vi "KDC101_Init.vi"(8 "error in (no error)":errorcluster caption="entrée d'erreur (pas d'erreur)", 11 "serialNo":string) -> (0 "error out":errorcluster caption="sortie d'erreur", 1 "Connected":bool, 2 "DevManRef":refnum<k24>, 3 "KCubeDCServoRef":refnum<k24>, 4 "SpeedSettings":T1, 5 "IsHomed":bool)   [LabVIEW 2019]
doc: "Utilisez ce modèle pour construire un VI à utiliser en tant que sous-VI."
uses:
  C:/Program Files (x86)/National Instruments/LabVIEW 2019/user.lib/ThorKDC101/Kinesis_with_LabVIEW_Examples_LV12 - v3/Thorlabs.MotionControl.DeviceManagerCLI.dll
  Kinesis_with_LabVIEW_Examples_LV12 - v3/Thorlabs.MotionControl.DeviceManagerCLI.dll
  C:/Program Files (x86)/National Instruments/LabVIEW 2019/user.lib/ThorKDC101/Kinesis_with_LabVIEW_Examples_LV12 - v3/ThorLabs.MotionControl.KCube.DCServoCLI.dll
  Kinesis_with_LabVIEW_Examples_LV12 - v3/ThorLabs.MotionControl.KCube.DCServoCLI.dll
  C:/Program Files (x86)/National Instruments/LabVIEW 2019/user.lib/ThorKDC101/Kinesis_with_LabVIEW_Examples_LV12 - v3/Thorlabs.MotionControl.GenericMotorCLI.dll
  Kinesis_with_LabVIEW_Examples_LV12 - v3/Thorlabs.MotionControl.GenericMotorCLI.dll
panel:
  out "MinVelocity":dbl
  out "MaxVelocity":dbl
  out "Acceleration":dbl
  out "array":string[](array[string])=["", "", "", "", "", "", "", "", "", "", " "]
  out "Capacity":i32
  out "Count":i32
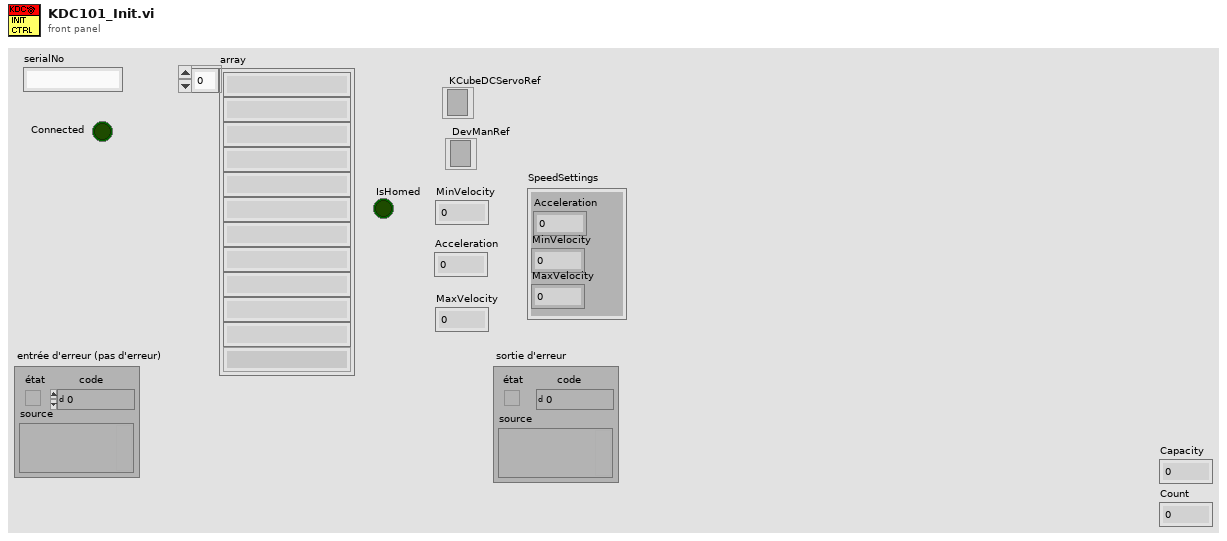
[diagram p1: front panel]
types:
  T1 = cluster{"Acceleration":dbl, "MinVelocity":dbl, "MaxVelocity":dbl}
  T2 = cluster{"Acceleration":dbl, "MaxVelocity":dbl, "MinVelocity":dbl}
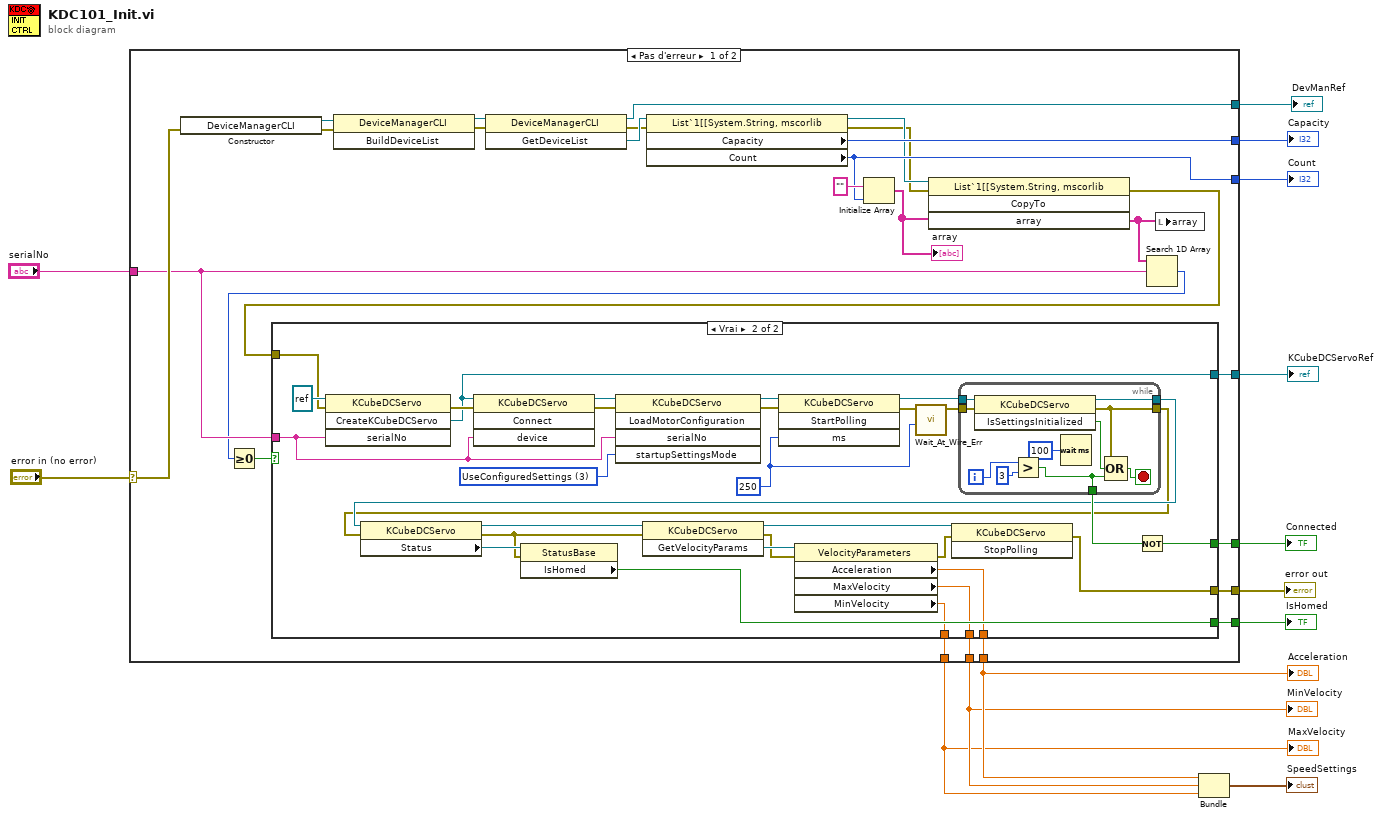
[diagram p0: block diagram]
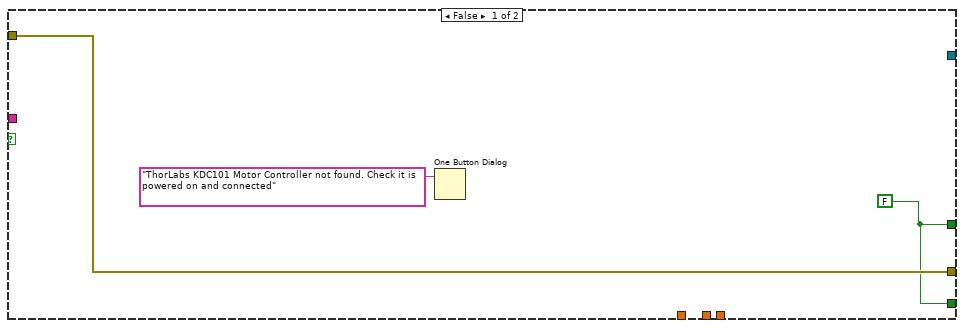
[diagram p2: hidden frame]
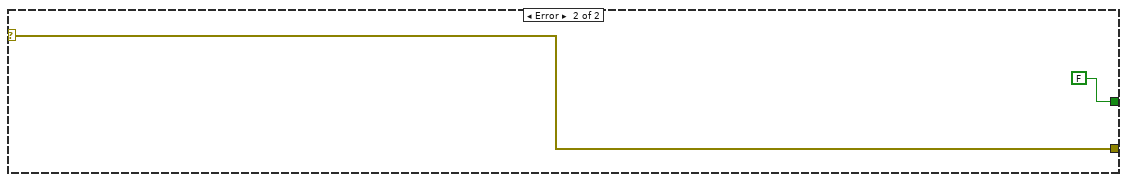
[diagram p3: hidden frame]
diagram:
  n1 = case shown="Pas d'erreur" "error in (no error)" {
    selector: "error in (no error)" -> [w36 w84]
    tunnel: [w18 w84] -> w12
    tunnel: [w33 _] -> w11
    tunnel: [w32 _] -> w10
    tunnel: [w30 _] -> w9
    tunnel: "serialNo" -> [w24 _]
    tunnel: [w23 _] -> w7
    tunnel: [w20 FALSE] -> w6
    tunnel: [w17 _] -> w5
    tunnel: [w16 _] -> w4
    tunnel: [w15 _] -> w3
    tunnel: [w14 _] -> w2
    frame No Error {
      n2 = constructor class="DeviceManagerCLI"(error in=w36) -> (reference out=w39:refnum<k24>, error out=w35:errorcluster)  [unwired: 2 in, 1 out]
      n3 = invoke class="DeviceManagerCLI" method="BuildDeviceList"(reference=w39, error in=w35) -> (reference out=w37:refnum<k24>, error out=w38:errorcluster)  [unwired: 1 in, 1 out]
      n4 = invoke class="DeviceManagerCLI" method="GetDeviceList"(reference=w37, error in=w38) -> (reference out=w30:refnum<k24>, error out=w29:errorcluster, "GetDeviceList"=w31:refnum<k24>)  [unwired: 1 in]
      n5 = property class="List`1[[System.String, mscorlib"(reference=w31, error in=w29) -> (reference out=w27:refnum<k24>, error out=w26:errorcluster, "Capacity"=w33:i32, "Count"=w32:i32)
      n6 = Initialize Array("", w32) -> (w28:string[])
      "array" <- w28
      n7 = invoke class="List`1[[System.String, mscorlib" method="CopyTo"(reference=w27, error in=w26, "array"=w28) -> (error out=w19:errorcluster, "array"=w25:string[])  [unwired: 1 in, 2 out]
      n8 = Search 1D Array(1D array=w25, element=w24) -> (index of element=w21:i32)  [unwired: 1 in]
      n9 = Greater Or Equal To 0?(x=w21) -> (x >= 0?=w22:bool)
      n10 = case shown="Vrai" w22 {
        tunnel: w24 -> [_ w67]
        tunnel: [_ w66] -> w23
        tunnel: [w40 w64] -> w20
        tunnel: w19 -> [w42 w63]
        tunnel: [w42 w46] -> w18
        tunnel: [w40 w49] -> w17
        tunnel: [_ w45] -> w16
        tunnel: [_ w44] -> w15
        tunnel: [_ w43] -> w14
        frame False {
          w40 = FALSE
          n11 = One Button Dialog(message="ThorLabs KDC101 Motor Controller not found. Check it is powered on and connected") -> ()  [unwired: 1 in, 1 out]
        }
        frame True {
          w57 = 250 ("ms")
          w70 = 3 items=["UseDeviceSettings"=1, "UseFileSettings"=2, "UseConfiguredSettings"=3] ("startupSettingsMode")
          n12 = invoke class="KCubeDCServo" method="CreateKCubeDCServo"(reference=refnum<k24> refnum ("target class"), error in=w63, "serialNo"=w67) -> (error out=w71:errorcluster, "CreateKCubeDCServo"=w66:refnum<k24>)  [unwired: 1 in, 2 out]
          n13 = invoke class="KCubeDCServo" method="Connect"(reference=w66, error in=w71, "device"=w67) -> (reference out=w69:refnum<k24>, error out=w68:errorcluster)  [unwired: 1 in, 2 out]
          n14 = invoke class="KCubeDCServo" method="LoadMotorConfiguration"(reference=w69, error in=w68, "serialNo"=w67, "startupSettingsMode"=w70) -> (reference out=w61:refnum<k24>, error out=w62:errorcluster)  [unwired: 1 in, 3 out]
          n15 = invoke class="KCubeDCServo" method="StartPolling"(reference=w61, error in=w62, "ms"=w57) -> (reference out=w60:refnum<k24>, error out=w59:errorcluster)  [unwired: 1 in, 2 out]
          n16 = call <userlib>:"Wait_At_Wire_Err.vi"("Wait (ms)"=w57, "error in (no error)"=w59) -> ("error out"=w58:errorcluster)  [unwired: 7 in, 2 out]
          n17 = while {
            tunnel: w60 -> [w82]
            tunnel: w58 -> [w74]
            tunnel: [w76] -> w65
            tunnel: [w75] -> w52
            tunnel: [w73] -> w53
            i -> [w79]
            stop <- w81 stop-if-true
            n18 = invoke class="KCubeDCServo" method="IsSettingsInitialized"(reference=w82, error in=w74) -> (reference out=w73:refnum<k24>, error out=w75:errorcluster, "IsSettingsInitialized"=w80:bool)  [unwired: 1 in]
            n19 = Greater?(x=w79, y=3) -> (0:w76:bool)
            n20 = Wait (ms)(milliseconds to wait=u32 100 ("attente (ms)")) -> ()  [unwired: 1 out]
            n21 = Compound Arithmetic op=OR ("Opérateur arithmétique")(w75, w80, w76) -> (w81:bool)
          }
          n22 = property class="KCubeDCServo"(reference=w53, error in=w52) -> (reference out=w55:refnum<k24>, error out=w54:errorcluster, "Status"=w56:refnum<k24>)
          n23 = property class="StatusBase"(reference=w56, error in=w54) -> ("IsHomed"=w49:bool)  [unwired: 2 out]
          n24 = invoke class="KCubeDCServo" method="GetVelocityParams"(reference=w55, error in=w54) -> (reference out=w47:refnum<k24>, error out=w50:errorcluster, "GetVelocityParams"=w51:refnum<k24>)  [unwired: 1 in]
          n25 = property class="VelocityParameters"(reference=w51, error in=w50) -> (error out=w48:errorcluster, "Acceleration"=w45:dbl, "MaxVelocity"=w44:dbl, "MinVelocity"=w43:dbl)  [unwired: 1 out]
          n26 = invoke class="KCubeDCServo" method="StopPolling"(reference=w47, error in=w48) -> (error out=w46:errorcluster)  [unwired: 1 in, 2 out]
          n27 = Not(x=w65) -> (.not. x?=w64:bool)
        }
      }
      n28 = local write "array"(w25) -> ()
    }
    frame Error {
    }
  }
  "error out" <- w12
  "Capacity" <- w11
  "Count" <- w10
  "DevManRef" <- w9
  "KCubeDCServoRef" <- w7
  "Connected" <- w6
  "IsHomed" <- w5
  "Acceleration" <- w4
  "MinVelocity" <- w3
  "MaxVelocity" <- w2
  n29 = Bundle("Acceleration"=w4, "MaxVelocity"=w3, "MinVelocity"=w2) -> (→"SpeedSettings":T2)  [unwired: 1 in]
